vi "main.vi"() -> ()   [LabVIEW 2015]
uses:
  Stany_enum.ctl
  <vilib>/DAQmx/write.llb/DAQmx Write (Analog Wfm 1Chan NSamp).vi
  <vilib>/DAQmx/read.llb/DAQmx Read (Analog 1D DBL 1Chan NSamp).vi
  <vilib>/DAQmx/create/channels.llb/DAQmx Create Channel (AO-Voltage-Basic).vi
  <vilib>/DAQmx/configure/timing.llb/DAQmx Timing (Use Waveform).vi
  <vilib>/DAQmx/miscellaneous.llb/DAQmx Fill In Error Info.vi
  <vilib>/DAQmx/create/channels.llb/DAQmx Create Channel (AI-Voltage-Basic).vi
  <vilib>/DAQmx/configure/timing.llb/DAQmx Timing (Sample Clock).vi
  <resource>/objmgr/daqmx.rc
panel:
  in  "Sterowanie\naplikacją":cluster{"Start pomiaru":bool, "Stop":bool}
  out "Ostatni błąd":errorcluster
  in  "Ustawienia\npomiaru":T1={"Kanal pomiaru"="", "Czestotliwosc pomiaru"=1000.0, "Liczba probek na kanal pomiarowy"=1000} {"Czestotliwosc pomiaru" format="%0.2f"}
  in  "Ustawienia\ngeneratora":T2={"Kanal generatora"="", "Ksztalt sygnalu"=enum."Sine Wave", "RegenMode"=10097} {"RegenMode" items=["Allow Regeneration"=10097, "Do Not Allow Regeneration"=10158]}
  out "Generowany sygnal":waveform(dbl)(graph)
  out "Pomiar":dbl[](graph)
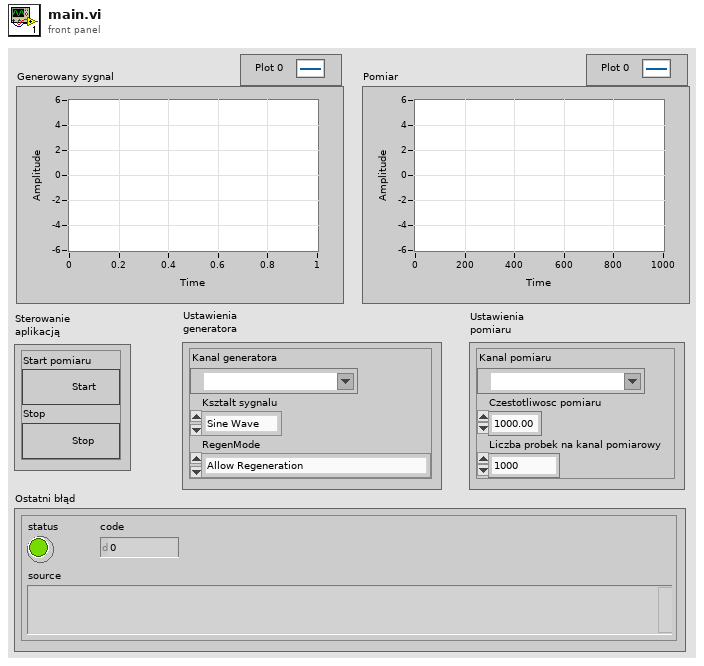
[diagram p1: front panel]
types:
  T1 = cluster{"Kanal pomiaru":tag, "Czestotliwosc pomiaru":dbl, "Liczba probek na kanal pomiarowy":i32}
  T2 = cluster{"Kanal generatora":tag, "Ksztalt sygnalu":enum16{"Sine Wave", "Triangle Wave", "Square Wave", "Sawtooth Wave"}, "RegenMode":i32}
  T3 = typedef "Stany_enum.ctl" = enum16{"Sprawdz czy STOP", "Czekaj na START", "Init", "Pracuj", "STOP", "Blad"}
  T4 = cluster{"RegenMode":refnum<vi>, "Ksztalt sygnalu":refnum<vi>, "Liczba probek na kanal pomiarowy":refnum<vi>, "Czestotliwosc pomiaru":refnum<vi>, "Kanal pomiaru":refnum<vi>, "Kanal generatora":refnum<vi>}
  T5 = enum8{"Enabled", "Disabled", "Disabled and Grayed Out"}
  T6 = enum16{"Sine Wave", "Triangle Wave", "Square Wave", "Sawtooth Wave"}
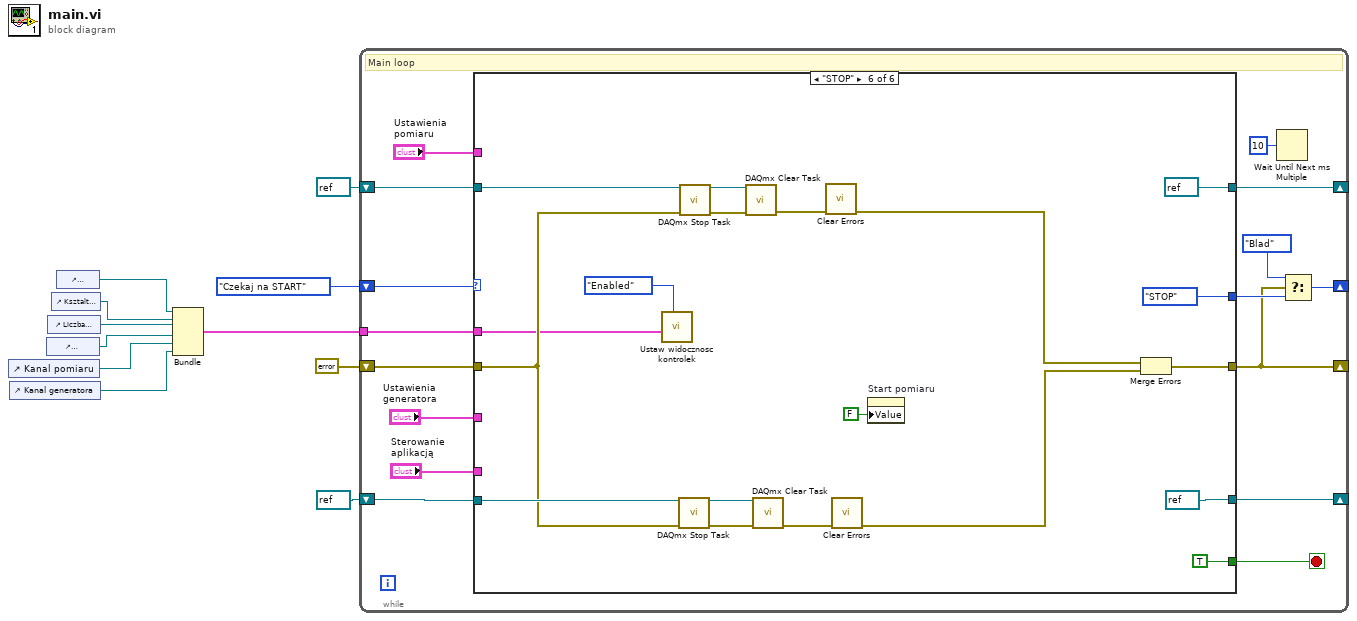
[diagram p0: block diagram]
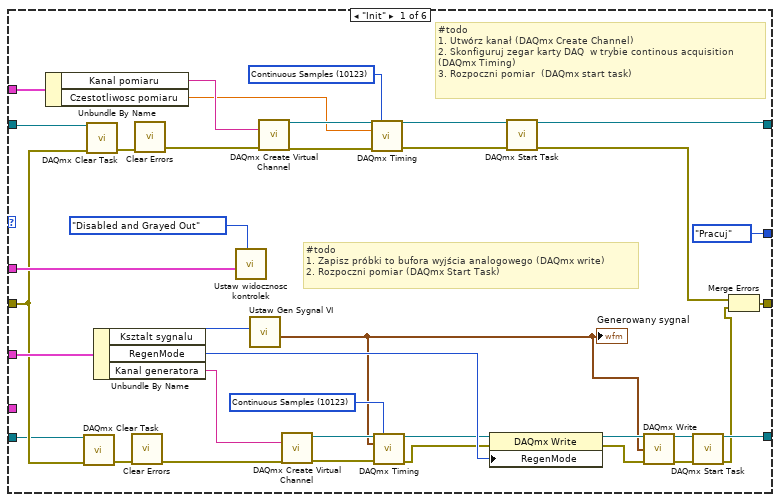
[diagram p2: hidden frame]
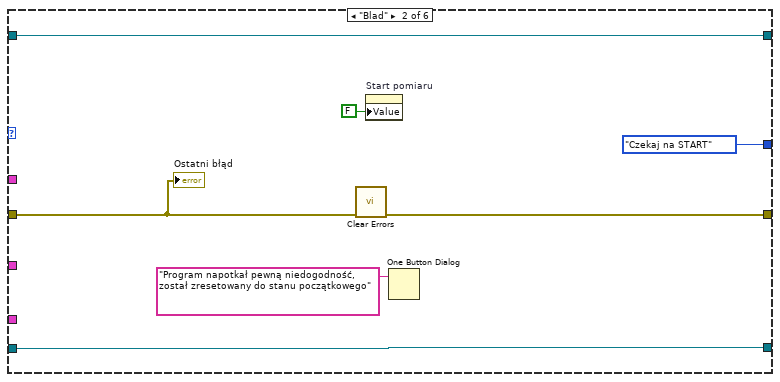
[diagram p3: hidden frame]
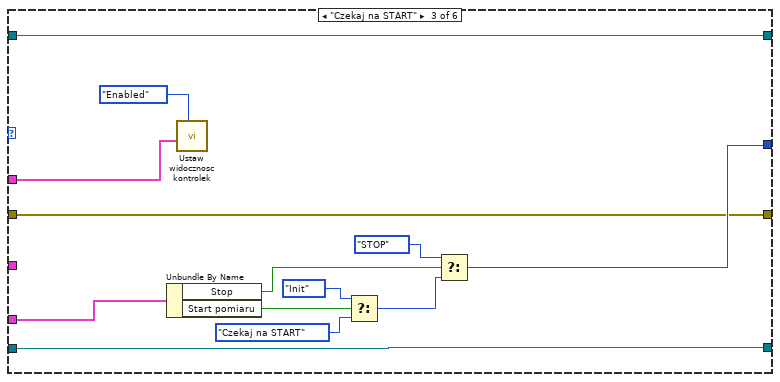
[diagram p4: hidden frame]
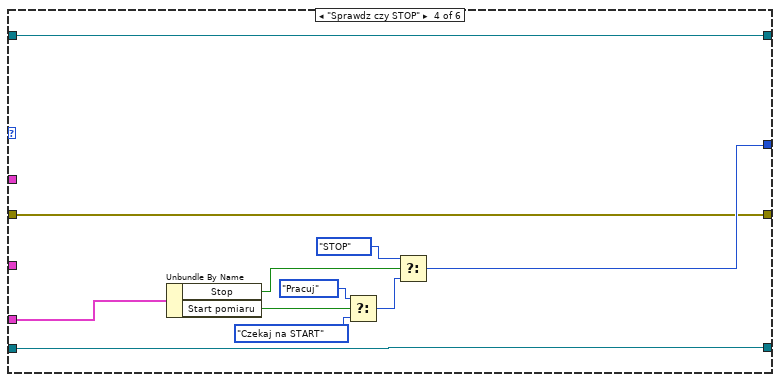
[diagram p5: hidden frame]
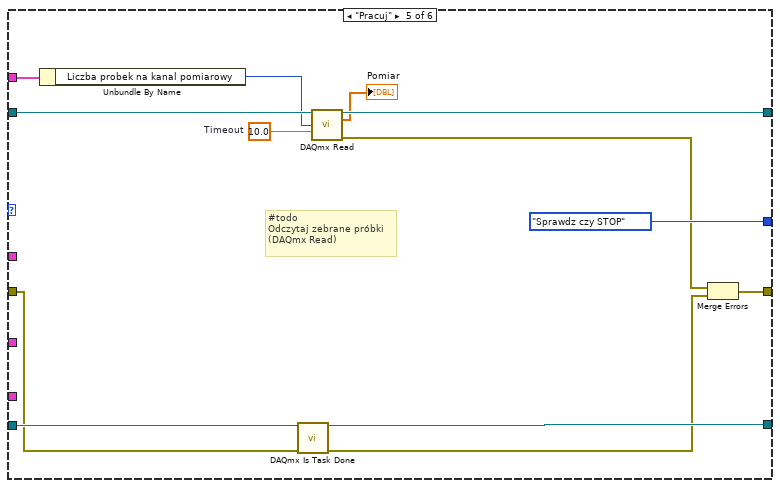
[diagram p6: hidden frame]
diagram:
  n1 = control-ref of="Kanal pomiaru"() -> (w3:refnum<vi>)
  n2 = control-ref of="Kanal generatora"() -> (w2:refnum<vi>)
  n3 = control-ref of="Czestotliwosc pomiaru"() -> (w4:refnum<vi>)
  n4 = control-ref of="Liczba probek na kanal pomiarowy"() -> (w5:refnum<vi>)
  n5 = control-ref of="Ksztalt sygnalu"() -> (w6:refnum<vi>)
  n6 = control-ref of="RegenMode"() -> (w7:refnum<vi>)
  n7 = Bundle("RegenMode"=w7, "Ksztalt sygnalu"=w6, "Liczba probek na kanal pomiarowy"=w5, "Czestotliwosc pomiaru"=w4, "Kanal pomiaru"=w3, "Kanal generatora"=w2) -> (w1:T4)  [unwired: 1 in]
  n8 = while {
    shift-right: [w26] -> _
    shift-left: refnum<k21> refnum ("task out") -> [w24]
    shift-right: [w25] -> _
    shift-left: refnum<k21> refnum ("task out") -> [w23]
    shift-right: [w17] -> _
    shift-left: Stany_enum."Czekaj na START" -> [w27]
    shift-right: [w18] -> _
    shift-left: errorcluster {"status"=FALSE, "code"=0, "source"=""} ("error out") -> [w20]
    tunnel: w1 -> [w12]
    stop <- w22 stop-if-true
    # "Main loop"
    n9 = case shown="\"STOP\"" w27 {
      tunnel: [w37 w70 w79 w86 w107 refnum<k21> refnum ("task out")] -> w26
      tunnel: [w30 w71 w80 w91 w105 refnum<k21> refnum ("task out")] -> w25
      tunnel: w24 -> [w49 w70 w79 w86 w108 w121]
      tunnel: w23 -> [w47 w71 w80 w91 w106 w118]
      tunnel: [Stany_enum."Pracuj" Stany_enum."Czekaj na START" w75 w87 Stany_enum."Sprawdz czy STOP" Stany_enum."STOP"] -> w19
      tunnel: [_ _ _ _ _ TRUE] -> w22
      tunnel: "Sterowanie\naplikacją" -> [_ _ w84 w95 _ _]
      tunnel: [w57 w69 w74 w85 w100 w113] -> w18
      tunnel: w20 -> [w48 w65 w74 w85 w101 w114]
      tunnel: "Ustawienia\ngeneratora" -> [w56 _ _ _ _ _]
      tunnel: "Ustawienia\npomiaru" -> [w55 _ _ _ w97 _]
      tunnel: w12 -> [w50 _ w73 _ _ w110]
      frame "Init" {
        w63 = 10123 items=["Finite Samples"=10178, "Continuous Samples"=10123, "Hardware Timed Single Point"=12522] ("sample mode")
        w44 = 10123 items=["Finite Samples"=10178, "Continuous Samples"=10123, "Hardware Timed Single Point"=12522] ("sample mode")
        # "#todo\n1. Zapisz próbki to bufora wyjścia analogowego (DAQmx write)\n2. Rozpoczni pomiar (DAQmx Start Task)"
        # "#todo\n1. Utwórz kanał (DAQmx Create Channel)\n2. Skonfiguruj zegar karty DAQ  w trybie continous acquisition\n(DAQmx Timing)\n3. Rozpoczni pomiar  (DAQmx start task)"
        n10 = Unbundle By Name(w55) -> ("Kanal pomiaru"=w46:tag, "Czestotliwosc pomiaru"=w41:dbl)
        n11 = call <vilib>:"DAQmx Clear Task.vi"("task in"=w47, "error in"=w48) -> ("error out"=w59:errorcluster)  [unwired: 13 in]
        n12 = call <vilib>:"DAQmx Clear Task.vi"("task in"=w49, "error in"=w48) -> ("error out"=w60:errorcluster)  [unwired: 13 in]
        n13 = Unbundle By Name(w56) -> ("Ksztalt sygnalu"=w53:T6, "RegenMode"=w52:i32, "Kanal generatora"=w54:tag)
        n14 = call <vilib>:"Clear Errors.vi"("error in (no error)"=w59) -> ("error out"=w58:errorcluster)  [unwired: 5 in, 1 out]
        n15 = call <vilib>:"Clear Errors.vi"("error in (no error)"=w60) -> ("error out"=w45:errorcluster)  [unwired: 5 in, 1 out]
        n16 = call "Ustaw widocznosc kontrolek.vi"("Disabled/Enabled"=T5."Disabled and Grayed Out" ("Disabled"), "Klaster referencji"=w50) -> ()  [unwired: 10 in]
        n17 = call "Ustaw Gen Sygnal VI.vi"("Ksztalt sygnalu"=w53) -> ("generowany sygnal"=w28:waveform(dbl))  [unwired: 10 in]
        "Generowany sygnal" <- w28
        n18 = call-poly <vilib>:"DAQmx Create Virtual Channel.vi"("physical channels"=w46, "error in"=w45) -> ("task out"=w43:refnum<k21>, "error out"=w42:errorcluster)  [unwired: 12 in]
        n19 = call-poly <vilib>:"DAQmx Create Virtual Channel.vi"("physical channels"=w54, "error in"=w58) -> ("task out"=w62:refnum<k21>, "error out"=w64:errorcluster)  [unwired: 12 in]
        n20 = call-poly <vilib>:"DAQmx Timing.vi"("task/channels in"=w43, "sample mode"=w44, "rate"=w41, "error in"=w42) -> ("task out"=w40:refnum<k21>, "error out"=w39:errorcluster)  [unwired: 10 in]
        n21 = call-poly <vilib>:"DAQmx Timing.vi"("task/channels in"=w62, "sample mode"=w63, "waveform"=w28, "error in"=w64) -> ("task out"=w36:refnum<k21>, "error out"=w35:errorcluster)  [unwired: 10 in]
        n22 = property class="DAQmx Write"(reference=w36, error in=w35, "RegenMode"=w52) -> (reference out=w32:refnum<k21>, error out=w31:errorcluster)
        n23 = call <vilib>:"DAQmx Start Task.vi"("task/channels in"=w40, "error in"=w39) -> ("task out"=w37:refnum<k21>, "error out"=w38:errorcluster)  [unwired: 12 in]
        n24 = call-poly <vilib>:"DAQmx Write.vi"("task/channels in"=w32, "data"=w28, "error in"=w31) -> ("task out"=w34:refnum<k21>, "error out"=w33:errorcluster)  [unwired: 10 in, 1 out]
        n25 = call <vilib>:"DAQmx Start Task.vi"("task/channels in"=w34, "error in"=w33) -> ("task out"=w30:refnum<k21>, "error out"=w29:errorcluster)  [unwired: 12 in]
        n26 = Merge Errors(w38, w29) -> (w57:errorcluster)
      }
      frame "Blad" {
        n27 = call <vilib>:"Clear Errors.vi"("error in (no error)"=w65) -> ("error out"=w69:errorcluster)  [unwired: 5 in, 1 out]
        n28 = property on="Start pomiaru" class="Bool (strict)"("Value"=FALSE) -> ()  [unwired: 2 in, 2 out]
        n29 = One Button Dialog(message="Program napotkał pewną niedogodność, został zresetowany do stanu początkowego") -> ()  [unwired: 1 in, 1 out]
        "Ostatni błąd" <- w65
      }
      frame "Czekaj na START" {
        n30 = Unbundle By Name(w84) -> ("Stop"=w78:bool, "Start pomiaru"=w83:bool)
        n31 = call "Ustaw widocznosc kontrolek.vi"("Disabled/Enabled"=T5."Enabled", "Klaster referencji"=w73) -> ()  [unwired: 10 in]
        n32 = Select(t=Stany_enum."Init", s=w83, f=Stany_enum."Czekaj na START") -> (s? t:f=w77:T3)
        n33 = Select(t=Stany_enum."STOP", s=w78, f=w77) -> (s? t:f=w75:T3)
      }
      frame "Sprawdz czy STOP" {
        n34 = Unbundle By Name(w95) -> ("Stop"=w90:bool, "Start pomiaru"=w94:bool)
        n35 = Select(t=Stany_enum."Pracuj", s=w94, f=Stany_enum."Czekaj na START") -> (s? t:f=w88:T3)
        n36 = Select(t=Stany_enum."STOP", s=w90, f=w88) -> (s? t:f=w87:T3)
      }
      frame "Pracuj" {
        w104 = 10.0  # Timeout
        # "#todo\nOdczytaj zebrane próbki\n(DAQmx Read)"
        n37 = Unbundle By Name(w97) -> ("Liczba probek na kanal pomiarowy"=w96:i32)
        n38 = call <vilib>:"DAQmx Is Task Done.vi"("task/channels in"=w106, "error in"=w101) -> ("task out"=w105:refnum<k21>, "error out"=w98:errorcluster)  [unwired: 11 in, 1 out]
        n39 = call-poly <vilib>:"DAQmx Read.vi"("task/channels in"=w108, "number of samples per channel"=w96, "timeout"=w104) -> ("task out"=w107:refnum<k21>, "data"=→"Pomiar":dbl[], "error out"=w99:errorcluster)  [unwired: 10 in]
        n40 = Merge Errors(w99, w98) -> (w100:errorcluster)
      }
      frame "STOP" {
        n41 = call "Ustaw widocznosc kontrolek.vi"("Disabled/Enabled"=T5."Enabled", "Klaster referencji"=w110) -> ()  [unwired: 10 in]
        n42 = call <vilib>:"DAQmx Stop Task.vi"("task/channels in"=w118, "error in"=w114) -> ("task out"=w119:refnum<k21>, "error out"=w120:errorcluster)  [unwired: 12 in]
        n43 = call <vilib>:"DAQmx Stop Task.vi"("task/channels in"=w121, "error in"=w114) -> ("task out"=w123:refnum<k21>, "error out"=w122:errorcluster)  [unwired: 12 in]
        n44 = call <vilib>:"DAQmx Clear Task.vi"("task in"=w123, "error in"=w122) -> ("error out"=w116:errorcluster)  [unwired: 13 in]
        n45 = call <vilib>:"DAQmx Clear Task.vi"("task in"=w119, "error in"=w120) -> ("error out"=w115:errorcluster)  [unwired: 13 in]
        n46 = call <vilib>:"Clear Errors.vi"("error in (no error)"=w116) -> ("error out"=w112:errorcluster)  [unwired: 5 in, 1 out]
        n47 = call <vilib>:"Clear Errors.vi"("error in (no error)"=w115) -> ("error out"=w111:errorcluster)  [unwired: 5 in, 1 out]
        n48 = property on="Start pomiaru" class="Bool (strict)"("Value"=FALSE ("Start pomiaru")) -> ()  [unwired: 2 in, 2 out]
        n49 = Merge Errors(w112, w111) -> (w113:errorcluster)
      }
    }
    n50 = Wait Until Next ms Multiple(millisecond multiple=u32 10) -> ()  [unwired: 1 out]
    n51 = Select(t=Stany_enum."Blad", s=w18, f=w19) -> (s? t:f=w17:T3)
  }
